vi "get_ctrl_refs.vi"(5 "vi_name":string, 6 "controls":string[](array[string])) -> (0 "error out":errorcluster, 1 "Controls[]":refnum<vi>[](array[refnum]))   [LabVIEW 2010]
panel:
  out "Array":string[](array[string])
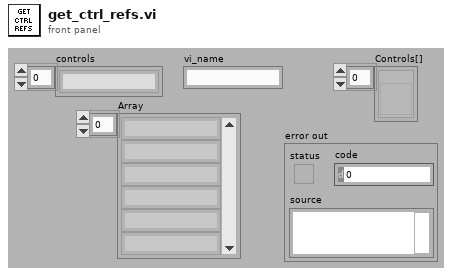
[diagram p1: front panel]
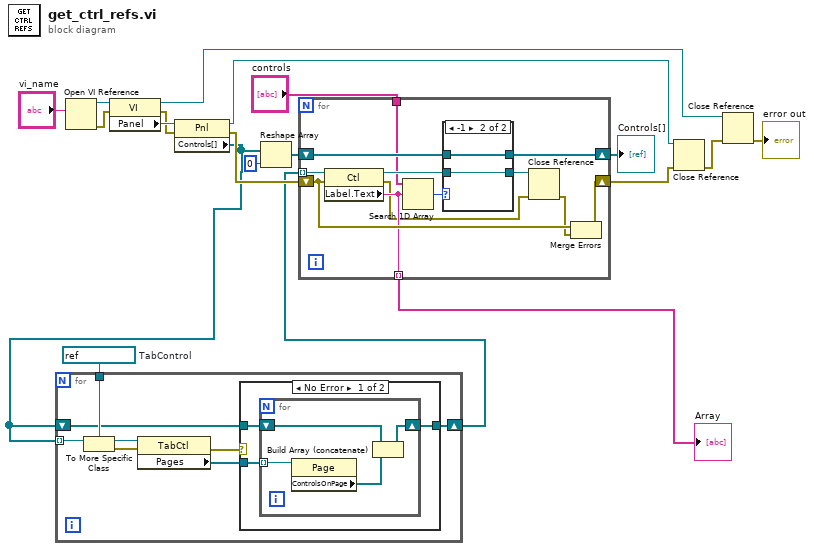
[diagram p0: block diagram]
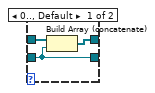
[diagram p3: hidden frame]
diagram:
  w4 = refnum<vi> refnum  # TabControl
  n1 = Open VI Reference(vi path="vi_name") -> (vi reference=w13:refnum<vi>, error out=w14:errorcluster)  [unwired: 5 in]
  n2 = property class="VI"(reference=w13, error in=w14) -> (reference out=w9:refnum<vi>, error out=w6:errorcluster, "Panel"=w15:refnum<vi>)
  n3 = property class="Pnl"(reference=w15, error in=w6) -> (reference out=w11:refnum<vi>, error out=w5:errorcluster, "Controls[]"=w1:refnum<vi>[])
  n4 = for {
    tunnel: w1 -> [w26] mode=indexing
    tunnel: w4 -> [w24]
    shift-right: [w21] -> w3
    shift-left: w1 -> [w22]
    n5 = To More Specific Class(target class=w24, reference=w26) -> (specific class reference=w25:refnum<vi>, error out=w23:errorcluster)  [unwired: 1 in]
    n6 = property class="TabCtl"(reference=w25, error in=w23) -> (error out=w20:errorcluster, "Pages"=w27:refnum<vi>[])  [unwired: 1 out]
    n7 = case shown="No Error" w20 {
      tunnel: w27 -> [w30 _]
      tunnel: w22 -> [w29 w35]
      tunnel: [w28 w35] -> w21
      frame No Error {
        n8 = for {
          tunnel: w30 -> [w34] mode=indexing
          shift-right: [w33] -> w28
          shift-left: w29 -> [w32]
          n9 = property class="Page"(reference=w34) -> ("ControlsOnPage"=w31:refnum<vi>[])  [unwired: 1 in, 2 out]
          n10 = Build Array (concatenate)(w32, w31) -> (w33:refnum<vi>[])
        }
      }
      frame Error {
      }
    }
  }
  n11 = Reshape Array(w1, 0 ("dimension size")) -> (w16:refnum<vi>[])
  n12 = for {
    tunnel: w3 -> [w47] mode=indexing
    shift-right: [w44] -> w18
    shift-left: w16 -> [w43]
    tunnel: "controls" -> [w42]
    shift-right: [w41] -> w10
    shift-left: w5 -> [w40]
    tunnel: [w39] -> w2 mode=indexing
    n13 = property class="Ctl"(reference=w47, error in=w40) -> (reference out=w45:refnum<vi>, error out=w38:errorcluster, "Label.Text"=w39:string)
    n14 = Search 1D Array(1D array=w42, element=w39) -> (index of element=w46:i32)  [unwired: 1 in]
    n15 = case shown="-1" w46 {
      tunnel: w45 -> [w48 w51]
      tunnel: [w50 w52] -> w44
      tunnel: w43 -> [w49 w52]
      tunnel: [w48 w51] -> w36
      frame 0.., Default {
        n16 = Build Array (concatenate)(w49, w48) -> (w50:refnum<vi>[])
      }
      frame -1 {
      }
    }
    n17 = Close Reference(reference=w36, error in (no error)=w38) -> (error out=w37:errorcluster)
    n18 = Merge Errors(w40, w37) -> (w41:errorcluster)
  }
  "Controls[]" <- w18
  "Array" <- w2
  n19 = Close Reference(reference=w11, error in (no error)=w10) -> (error out=w8:errorcluster)
  n20 = Close Reference(reference=w9, error in (no error)=w8) -> (error out=→"error out":errorcluster)
